vi "ConfigureHardware.vi"(8 "error in (no error)":errorcluster, 11 "Scan Engine Config":T1) -> (0 "error out":errorcluster, 3 "Scan Engine Config out":T1)   [LabVIEW 2017, in "ScanEngine.lvlib"]
uses:
  <vilib>/addons/InsightCM/Devices/Shared/Common/ScanEngine/ScanEngine.lvlib
  <vilib>/addons/InsightCM/Devices/Shared/Common/ScanEngine/controls/Configuration.ctl
  <vilib>/addons/InsightCM/Devices/Shared/Common/ScanEngine/controls/Group.ctl
  <vilib>/addons/InsightCM/Devices/Shared/Common/ScanEngine/controls/Channel.ctl
  <vilib>/Utility/Data Type/Type Definitions/Data Type.ctl
  <vilib>/addons/InsightCM/MessageBus/Base/controls/KeyValuePair.ctl
  <vilib>/Utility/Data Type/NI_Data Type.lvlib
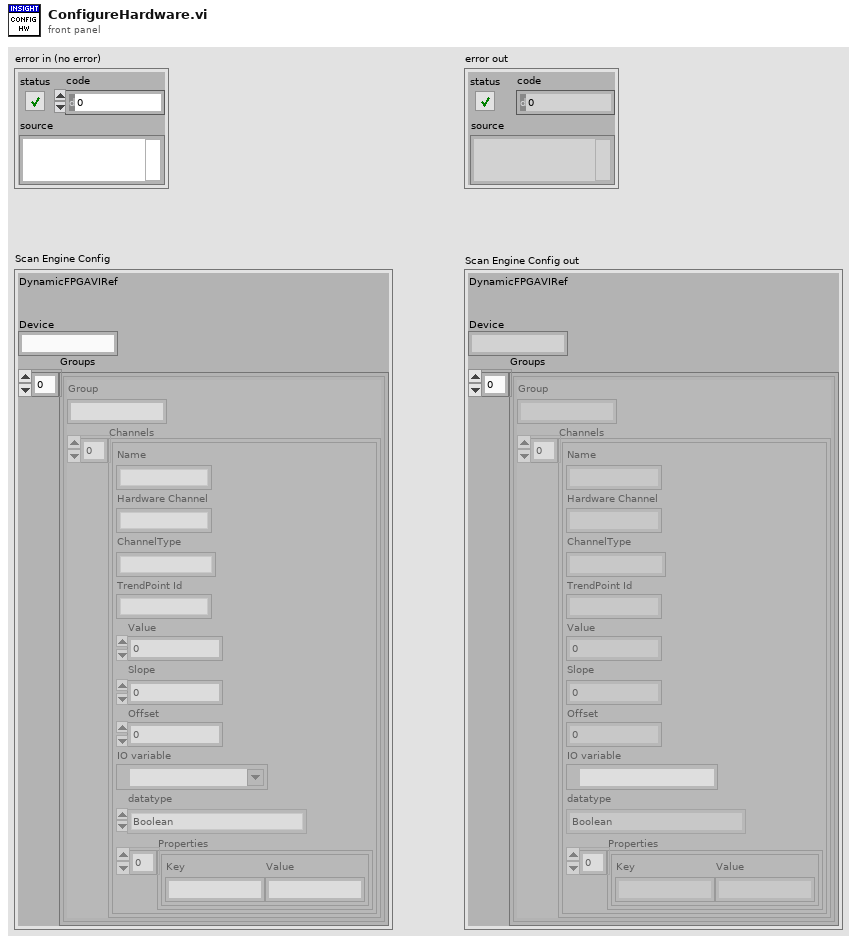
[diagram p1: front panel]
types:
  T1 = typedef "ScanEngine.lvlib/Configuration.ctl" = cluster{"DynamicFPGAVIRef":refnum<k20>, "Device":string, "Groups":T2[]}
  T2 = typedef "ScanEngine.lvlib/Group.ctl" = cluster{"Group":string, "Channels":T3[]}
  T3 = typedef "ScanEngine.lvlib/Channel.ctl" = cluster{"Name":string, "Hardware Channel":string, "ChannelType":string, "TrendPoint Id":string, "Value":sgl, "Slope":dbl, "Offset":dbl, "IO variable":refnum<k21>, "datatype":T4, "Properties":T5[]}
  T4 = typedef "NI_Data Type.lvlib/Data Type.ctl" = enum8{"Invalid Type", "Void", "I8", "I16", "I32", "I64", "U8", "U16", "U32", "U64", "Single Float", "Double Float", "Extended Float", "Single Complex", "Double Complex", "Extended Complex", "Enum U8", "Enum U16", "Enum U32", "Enum U64", "Single Float With Unit", "Double Float With Unit", "Extended Float With Unit", "Single Complex with Unit", "Double Complex with Unit", "Extended Complex with Unit", "Boolean", "String", "Path", "Picture", "Tag", "Array", "Cluster", "Variant", "LV Variant", "Waveform", "Timestamp", "Digital Waveform", "Digital Data", "ExpressData", "Refnum", "External Data", "VI", "Poly VI", "LabVIEW Class Instance", "Fixed Point"}
  T5 = typedef "KeyValuePair.ctl" = cluster{"Key":string, "Value":string}
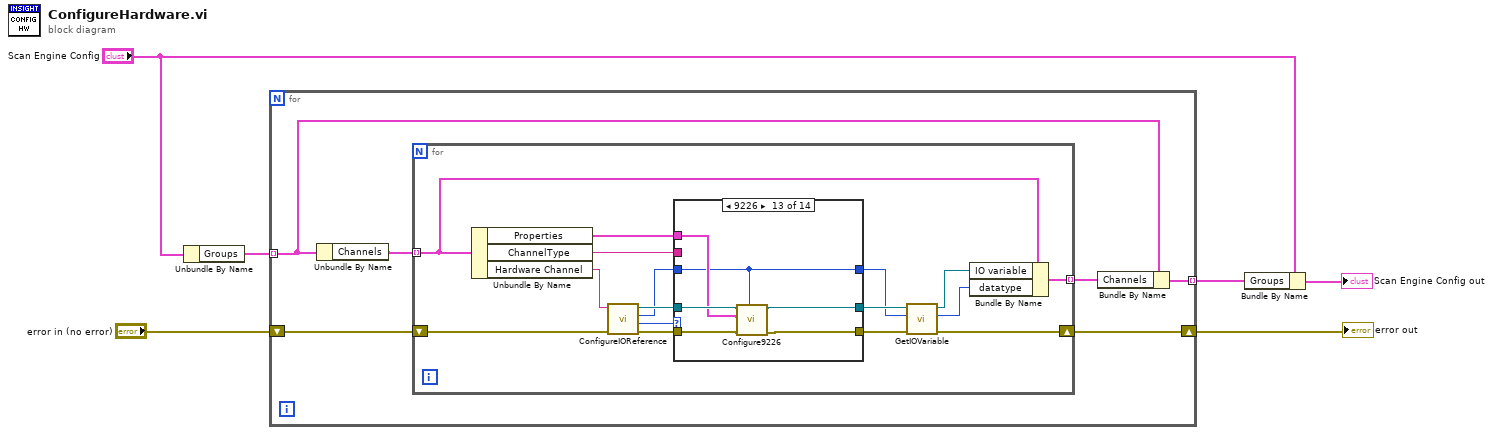
[diagram p0: block diagram]
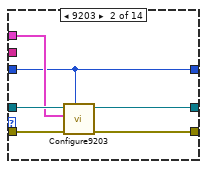
[diagram p3: hidden frame]
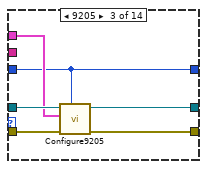
[diagram p4: hidden frame]
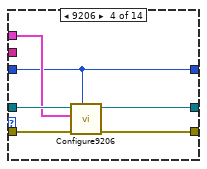
[diagram p5: hidden frame]
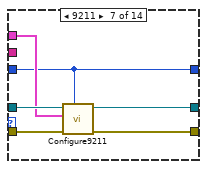
[diagram p8: hidden frame]
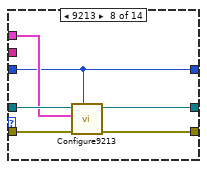
[diagram p9: hidden frame]
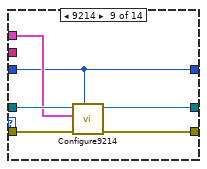
[diagram p10: hidden frame]
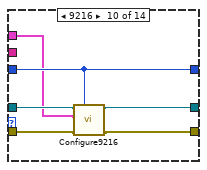
[diagram p11: hidden frame]
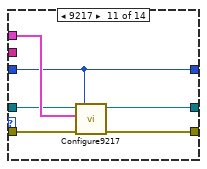
[diagram p12: hidden frame]
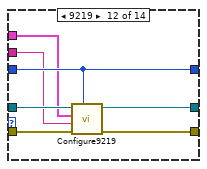
[diagram p13: hidden frame]
diagram:
  n1 = Unbundle By Name("Scan Engine Config") -> ("Groups"=w5:T2[])
  n2 = for {
    tunnel: w5 -> [w10] mode=indexing
    tunnel: [w8] -> w3 mode=indexing
    shift-right: [w7] -> w1
    shift-left: "error in (no error)" -> [w12]
    n3 = Unbundle By Name(w10) -> ("Channels"=w11:T3[])
    n4 = for {
      shift-right: [w19] -> w7
      shift-left: w12 -> [w28]
      tunnel: [w17] -> w9 mode=indexing
      tunnel: w11 -> [w13] mode=indexing
      n5 = Unbundle By Name(w13) -> ("Properties"=w16:T5[], "ChannelType"=w15:string, "Hardware Channel"=w21:string)
      n6 = call <vilib>:"ConfigureIOReference.vi"("error in (no error)"=w28, "Hardware Channel"=w21) -> ("error out"=w20:errorcluster, "Model"=w22:u32, "Channel Number"=w26:i32, "IO Ref"=w27:refnum<k21>)  [unwired: 6 in]
      n7 = case shown="9226" w22 {
        tunnel: w20 -> [w31 w37 w42 w48 w50 w55 w60 w67 w73 w76 w83 w91 w95 w101]
        tunnel: [w31 w34 w43 w49 w50 w55 w61 w65 w71 w75 w84 w92 w94 w101] -> w25
        tunnel: w26 -> [w30 w32 w38 w44 w51 w54 w56 w62 w68 w79 w80 w88 w93 w100]
        tunnel: w27 -> [w29 w36 w41 w47 w52 w53 w59 w66 w72 w78 w81 w90 w97 w99]
        tunnel: [w29 w35 w40 w46 w52 w53 w58 w64 w70 w74 w85 w89 w98 w99] -> w24
        tunnel: [w30 w32 w38 w44 w51 w54 w56 w62 w68 w79 w80 w88 w93 w100] -> w23
        tunnel: w16 -> [_ w33 w39 w45 _ _ w57 w63 w69 w77 w82 w87 w96 _]
        tunnel: w15 -> [_ _ _ _ _ _ _ _ _ _ _ w86 _ _]
        frame Default {
        }
        frame 9203 {
          n8 = call <vilib>:"Configure9203.vi"("Channel Number"=w32, "error in (no error)"=w37, "Properties"=w33, "IO Ref in"=w36) -> ("error out"=w34:errorcluster, "IO Ref out"=w35:refnum<k21>)  [unwired: 6 in]
        }
        frame 9205 {
          n9 = call <vilib>:"Configure9205.vi"("Channel Number"=w38, "error in (no error)"=w42, "Properties"=w39, "IO Ref"=w41) -> ("error out"=w43:errorcluster, "IO Ref out"=w40:refnum<k21>)  [unwired: 6 in]
        }
        frame 9206 {
          n10 = call <vilib>:"Configure9206.vi"("Channel Number"=w44, "error in (no error)"=w48, "Properties"=w45, "IO Ref in"=w47) -> ("error out"=w49:errorcluster, "IO Ref out"=w46:refnum<k21>)  [unwired: 6 in]
        }
        frame 9207 {
          # "no channel configuration"
        }
        frame 9208 {
          # "no channel configuration"
        }
        frame 9211 {
          n11 = call <vilib>:"Configure9211.vi"("Channel Number"=w56, "error in (no error)"=w60, "Properties"=w57, "Refnum in"=w59) -> ("error out"=w61:errorcluster, "Refnum out"=w58:refnum<k21>)  [unwired: 6 in]
        }
        frame 9213 {
          n12 = call <vilib>:"Configure9213.vi"("Channel Number"=w62, "error in (no error)"=w67, "Properties"=w63, "IO Ref in"=w66) -> ("error out"=w65:errorcluster, "IO Ref out"=w64:refnum<k21>)  [unwired: 6 in]
        }
        frame 9214 {
          n13 = call <vilib>:"Configure9214.vi"("Channel Number"=w68, "error in (no error)"=w73, "Properties"=w69, "IO Ref"=w72) -> ("error out"=w71:errorcluster, "IO Ref out"=w70:refnum<k21>)  [unwired: 6 in]
        }
        frame 9216 {
          n14 = call <vilib>:"Configure9216.vi"("Channel Number"=w79, "error in (no error)"=w76, "Properties"=w77, "IO Ref"=w78) -> ("error out"=w75:errorcluster, "IO Ref out"=w74:refnum<k21>)  [unwired: 6 in]
        }
        frame 9217 {
          n15 = call <vilib>:"Configure9217.vi"("Channel Number"=w80, "error in (no error)"=w83, "Properties"=w82, "IO Ref"=w81) -> ("error out"=w84:errorcluster, "IO Ref out"=w85:refnum<k21>)  [unwired: 6 in]
        }
        frame 9219 {
          n16 = call <vilib>:"Configure9219.vi"("Channel Number"=w88, "error in (no error)"=w91, "ChannelType"=w86, "Properties"=w87, "IO Ref in"=w90) -> ("error out"=w92:errorcluster, "IO Ref out"=w89:refnum<k21>)  [unwired: 5 in]
        }
        frame 9226 {
          n17 = call <vilib>:"Configure9226.vi"("Channel Number"=w93, "error in (no error)"=w95, "Properties"=w96, "IO Ref"=w97) -> ("error out"=w94:errorcluster, "IO Ref out"=w98:refnum<k21>)  [unwired: 6 in]
        }
        frame 9229, 9239 {
          # "no channel configuration"
        }
      }
      n18 = call <vilib>:"GetIOVariable.vi"("error in (no error)"=w25, "Channel Number"=w23, "IO Ref"=w24) -> ("error out"=w19:errorcluster, "Type"=w14:T4, "IO Variable Ref"=w18:refnum<k21>)  [unwired: 6 in]
      n19 = Bundle By Name(cluster=w13, "IO variable"=w18, "datatype"=w14) -> (w17:T3)
    }
    n20 = Bundle By Name(cluster=w10, "Channels"=w9) -> (w8:T2)
  }
  "error out" <- w1
  n21 = Bundle By Name(cluster="Scan Engine Config", "Groups"=w3) -> (→"Scan Engine Config out":T1)
